vi "CalcDifference.vi"(11 "DataIn":i32[](array[numeric])) -> (3 "DataOut":dbl[](array[numeric]))   [LabVIEW 2017]
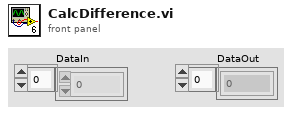
[diagram p1: front panel]
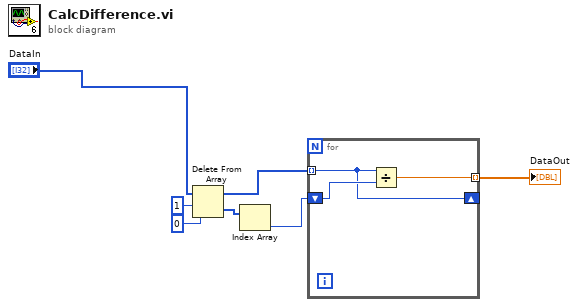
[diagram p0: block diagram]
diagram:
  n1 = Delete From Array(array="DataIn", length=1, index=0) -> (deleted portion=w3:i32[], array with subset deleted=w5:i32[])
  n2 = Index Array(array=w3) -> (element=w4:i32)  [unwired: 1 in]
  n3 = for {
    shift-right: [w9] -> _
    shift-left: w4 -> [w10]
    tunnel: w5 -> [w9] mode=indexing
    tunnel: [w8] -> w6 mode=indexing
    n4 = Divide(x=w9, y=w10) -> (x/y=w8:dbl)
  }
  "DataOut" <- w6
